vi "sedSpectrometer_logEvent_TimeOut.vi"(8 "error in (no error)":errorcluster, 11 "logevent_TimeOut_Ctl":T1) -> (0 "error out":errorcluster, 2 "function return":i32, 3 "logevent_TimeOut_Ctl out":T1)   [LabVIEW 2016, in "SALLV_sedSpectrometer.lvlib"]
doc: "int sedSpectrometer_shm_logEvent_TimeOutLV(sedSpectrometer_logevent_TimeOutLV *logevent_TimeOut_Ctl );"
uses:
  SALLV_sedSpectrometer.lvlib
  DataTypes/logevent_TimeOut.ctl
  SALLV_sedSpectrometer.so
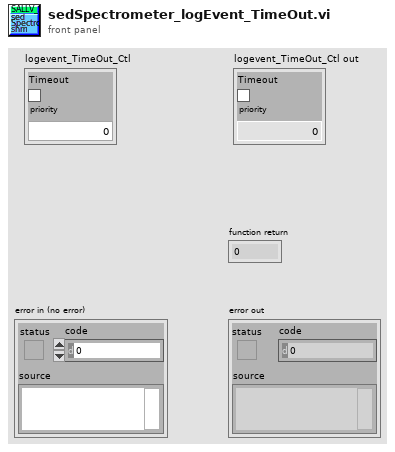
[diagram p1: front panel]
types:
  T1 = typedef "SALLV_sedSpectrometer.lvlib/logevent_TimeOut.ctl" = cluster{"Timeout":bool, "priority":i32}
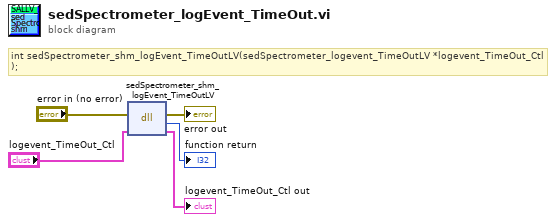
[diagram p0: block diagram]
diagram:
  # "int sedSpectrometer_shm_logEvent_TimeOutLV(sedSpectrometer_logevent_TimeOutLV *logevent_TimeOut_Ctl );"
  n1 = dll-call lib="home/harini/TCS/SALLV_sedSpectrometer/SALLV_sedSpectrometer.*" fn="sedSpectrometer_shm_logEvent_TimeOutLV"(error in="error in (no error)", "logevent_TimeOut_Ctl"="logevent_TimeOut_Ctl") -> (error out=→"error out":errorcluster, →"function return":i32, "logevent_TimeOut_Ctl"=→"logevent_TimeOut_Ctl out":T1)  [unwired: 2 in, 1 out]
